vi "Post_Refresh_Request.vi"(8 "error in (no error)":errorcluster, 11 "Asana in":refnum<class "Asana.lvclass">) -> (0 "error out":errorcluster, 3 "Asana out":refnum<class "Asana.lvclass">)   [LabVIEW 2016, in "Asana.lvclass"]
uses:
  Asana.lvclass
  OAuth/OAuth.lvclass
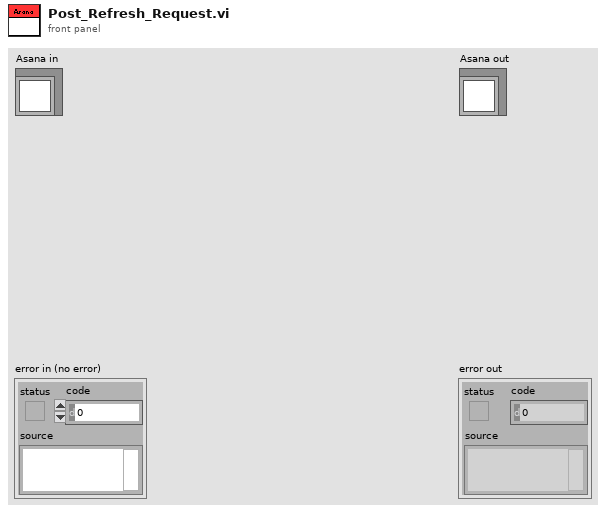
[diagram p1: front panel]
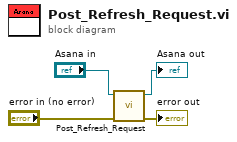
[diagram p0: block diagram]
diagram:
  n1 = call-parent "Post_Refresh_Request.vi"("error in (no error)"="error in (no error)", "OAuth in"="Asana in") -> ("error out"=→"error out":errorcluster, "OAuth out"=→"Asana out":refnum<class "Asana.lvclass">)  [unwired: 8 in]
